vi "vPR_translate.vi"(9 "資料表欄位名稱":string[](array[string]), 10 "欄位數":i32, 11 "Input":T1(array[cluster])) -> (3 "輸出資料":string[][](array[string]))   [LabVIEW 2019]
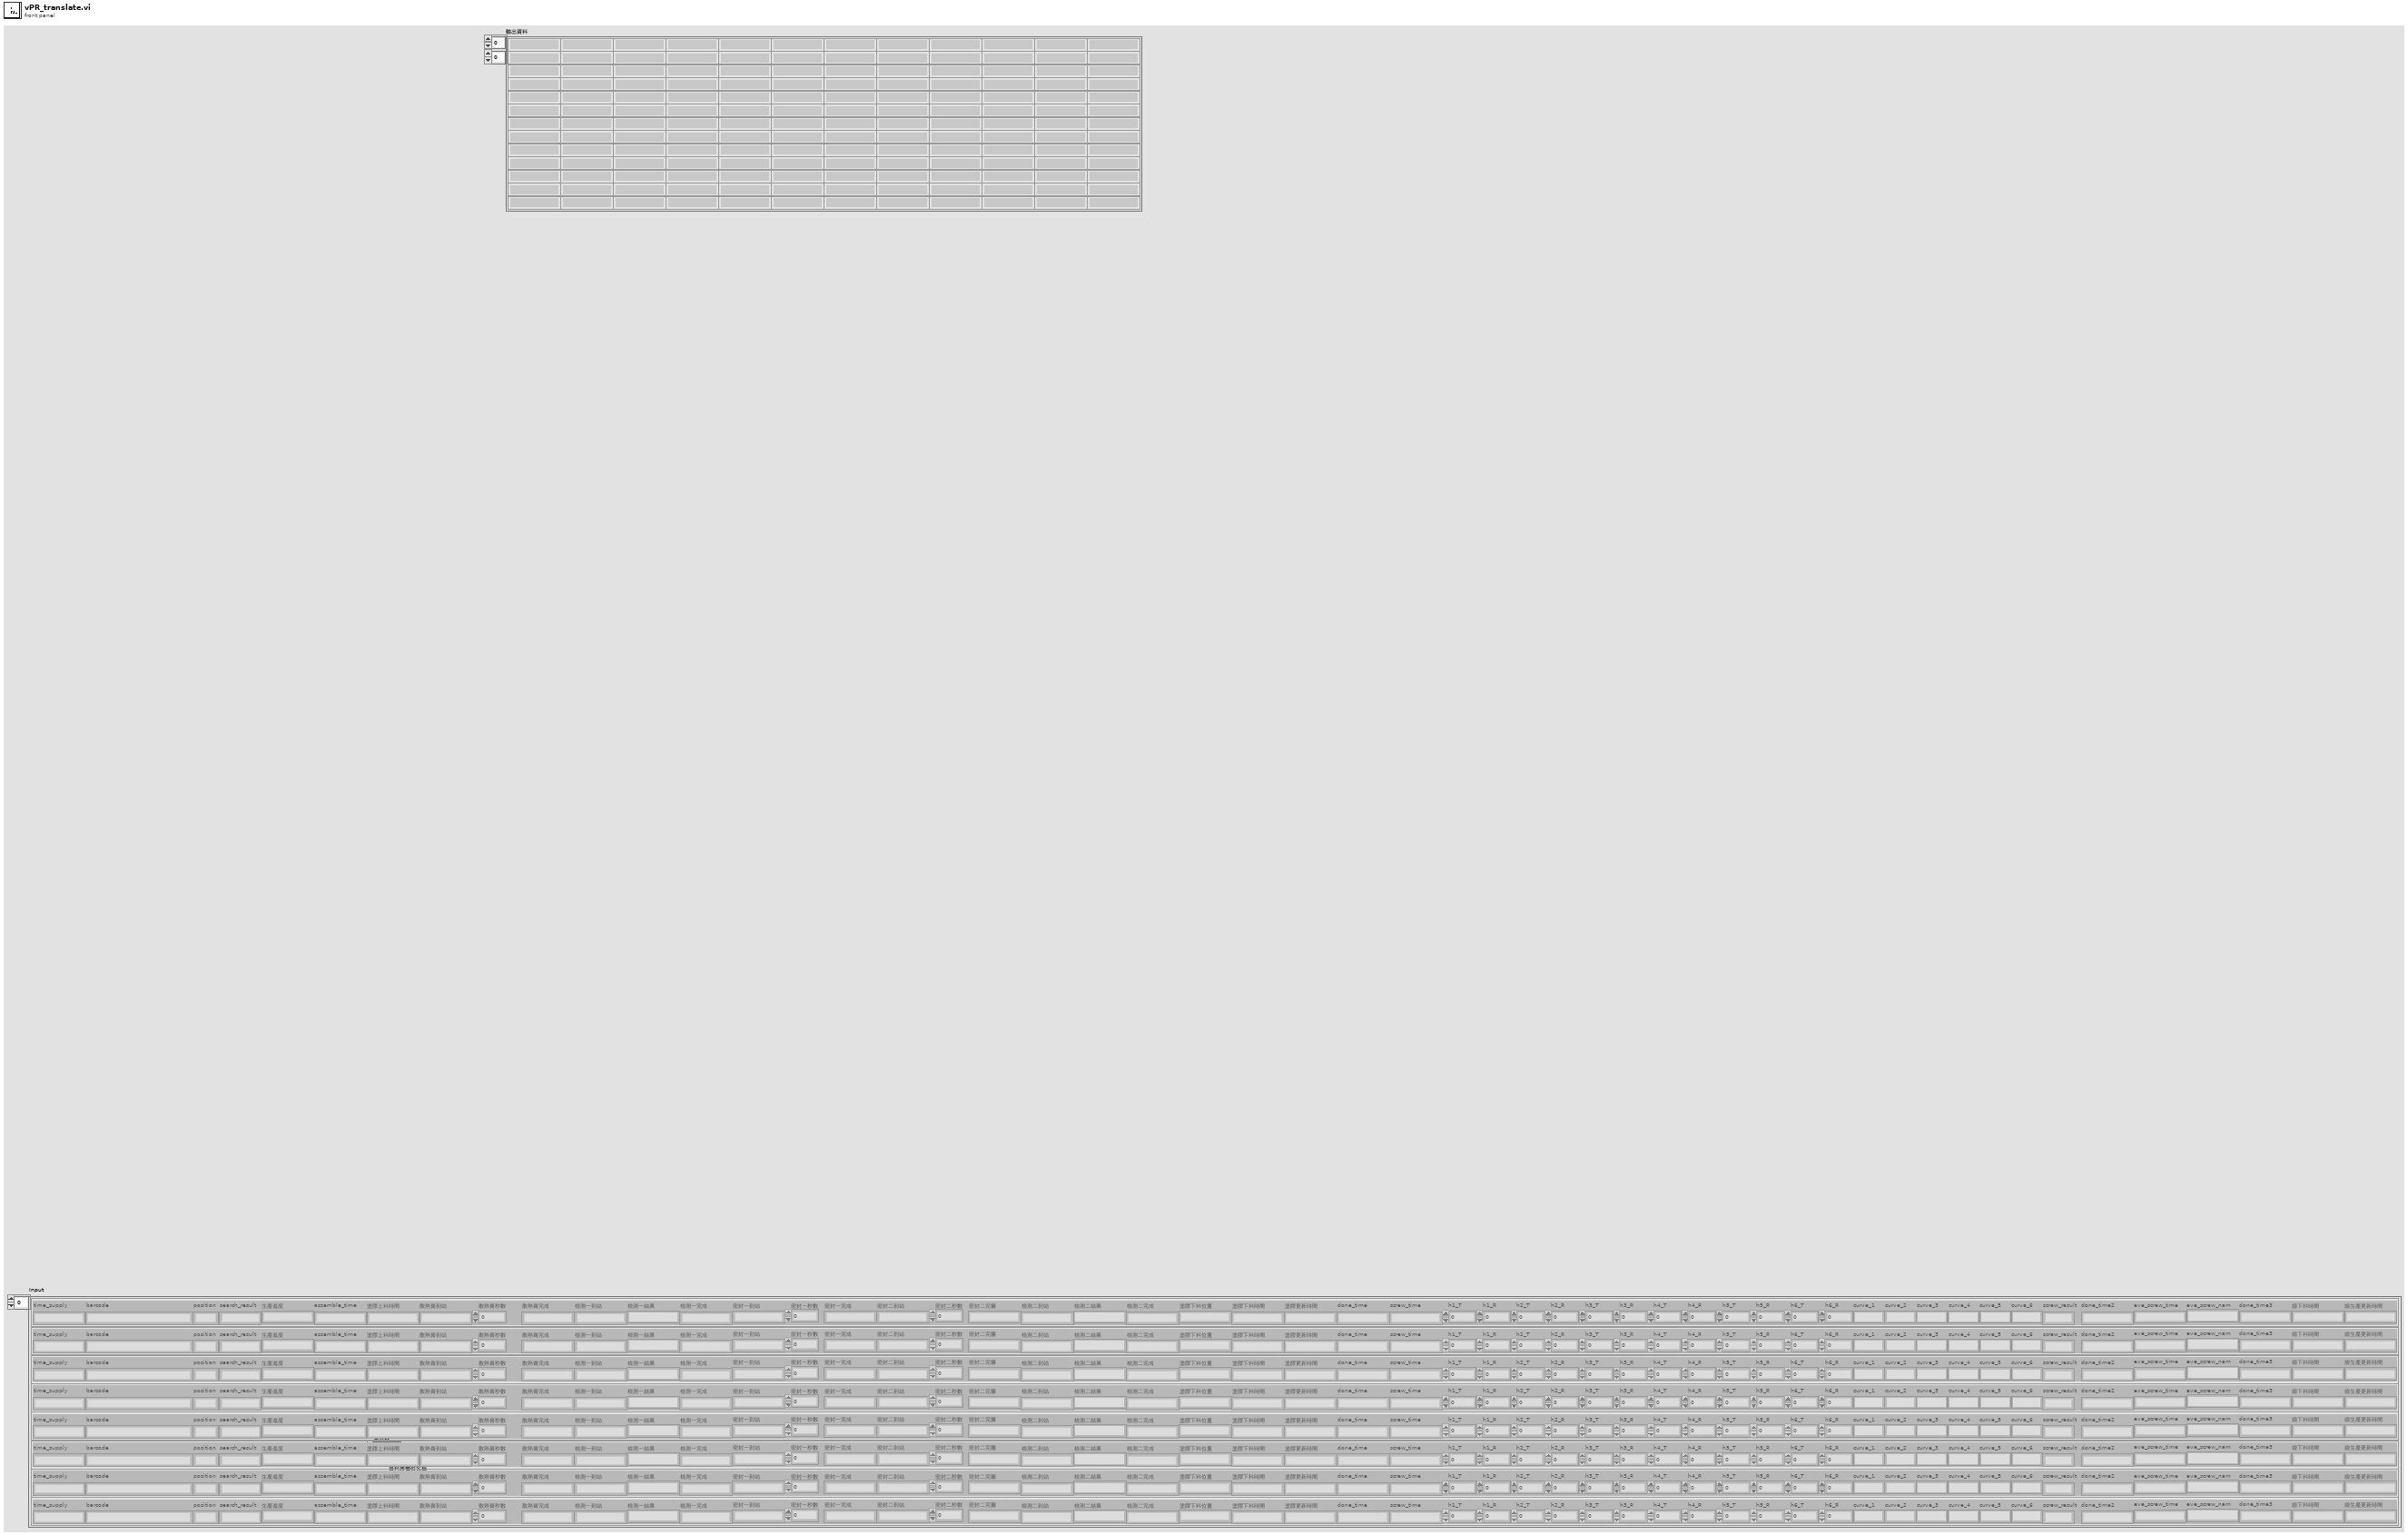
[diagram p1: front panel]
types:
  T1 = cluster{"time_supply":string, "barcode":string, "position":string, "search_result":string, "生產進度":string, "assemble_time":string, "塗膠上料時間":string, "散熱膏到站":string, "散熱膏秒數":dbl, "散熱膏完成":string, "檢測一到站":string, "檢測一結果":string, "檢測一完成":string, "密封一到站":string, "密封一秒數":dbl, "密封一完成":string, "密封二到站":string, "密封二秒數":dbl, "密封二完籌":string, "檢測二到站":string, "檢測二結果":string, "檢測二完成":string, "塗膠下料位置":string, "塗膠下料時間":string, "塗膠更新時間":string, "done_time":string, "screw_time":string, "h1_T":dbl, "h1_R":dbl, "h2_T":dbl, "h2_R":dbl, "h3_T":dbl, "h3_R":dbl, "h4_T":dbl, "h4_R":dbl, "h5_T":dbl, "h5_R":dbl, "h6_T":dbl, "h6_R":dbl, "curve_1":string, "curve_2":string, "curve_3":string, "curve_4":string, "curve_5":string, "curve_6":string, "screw_result":string, "done_time2":string, "eve_screw_time":string, "eve_screw_nam":string, "done_time3":string, "總下料時間":string, "總生產更新時間":string}[]
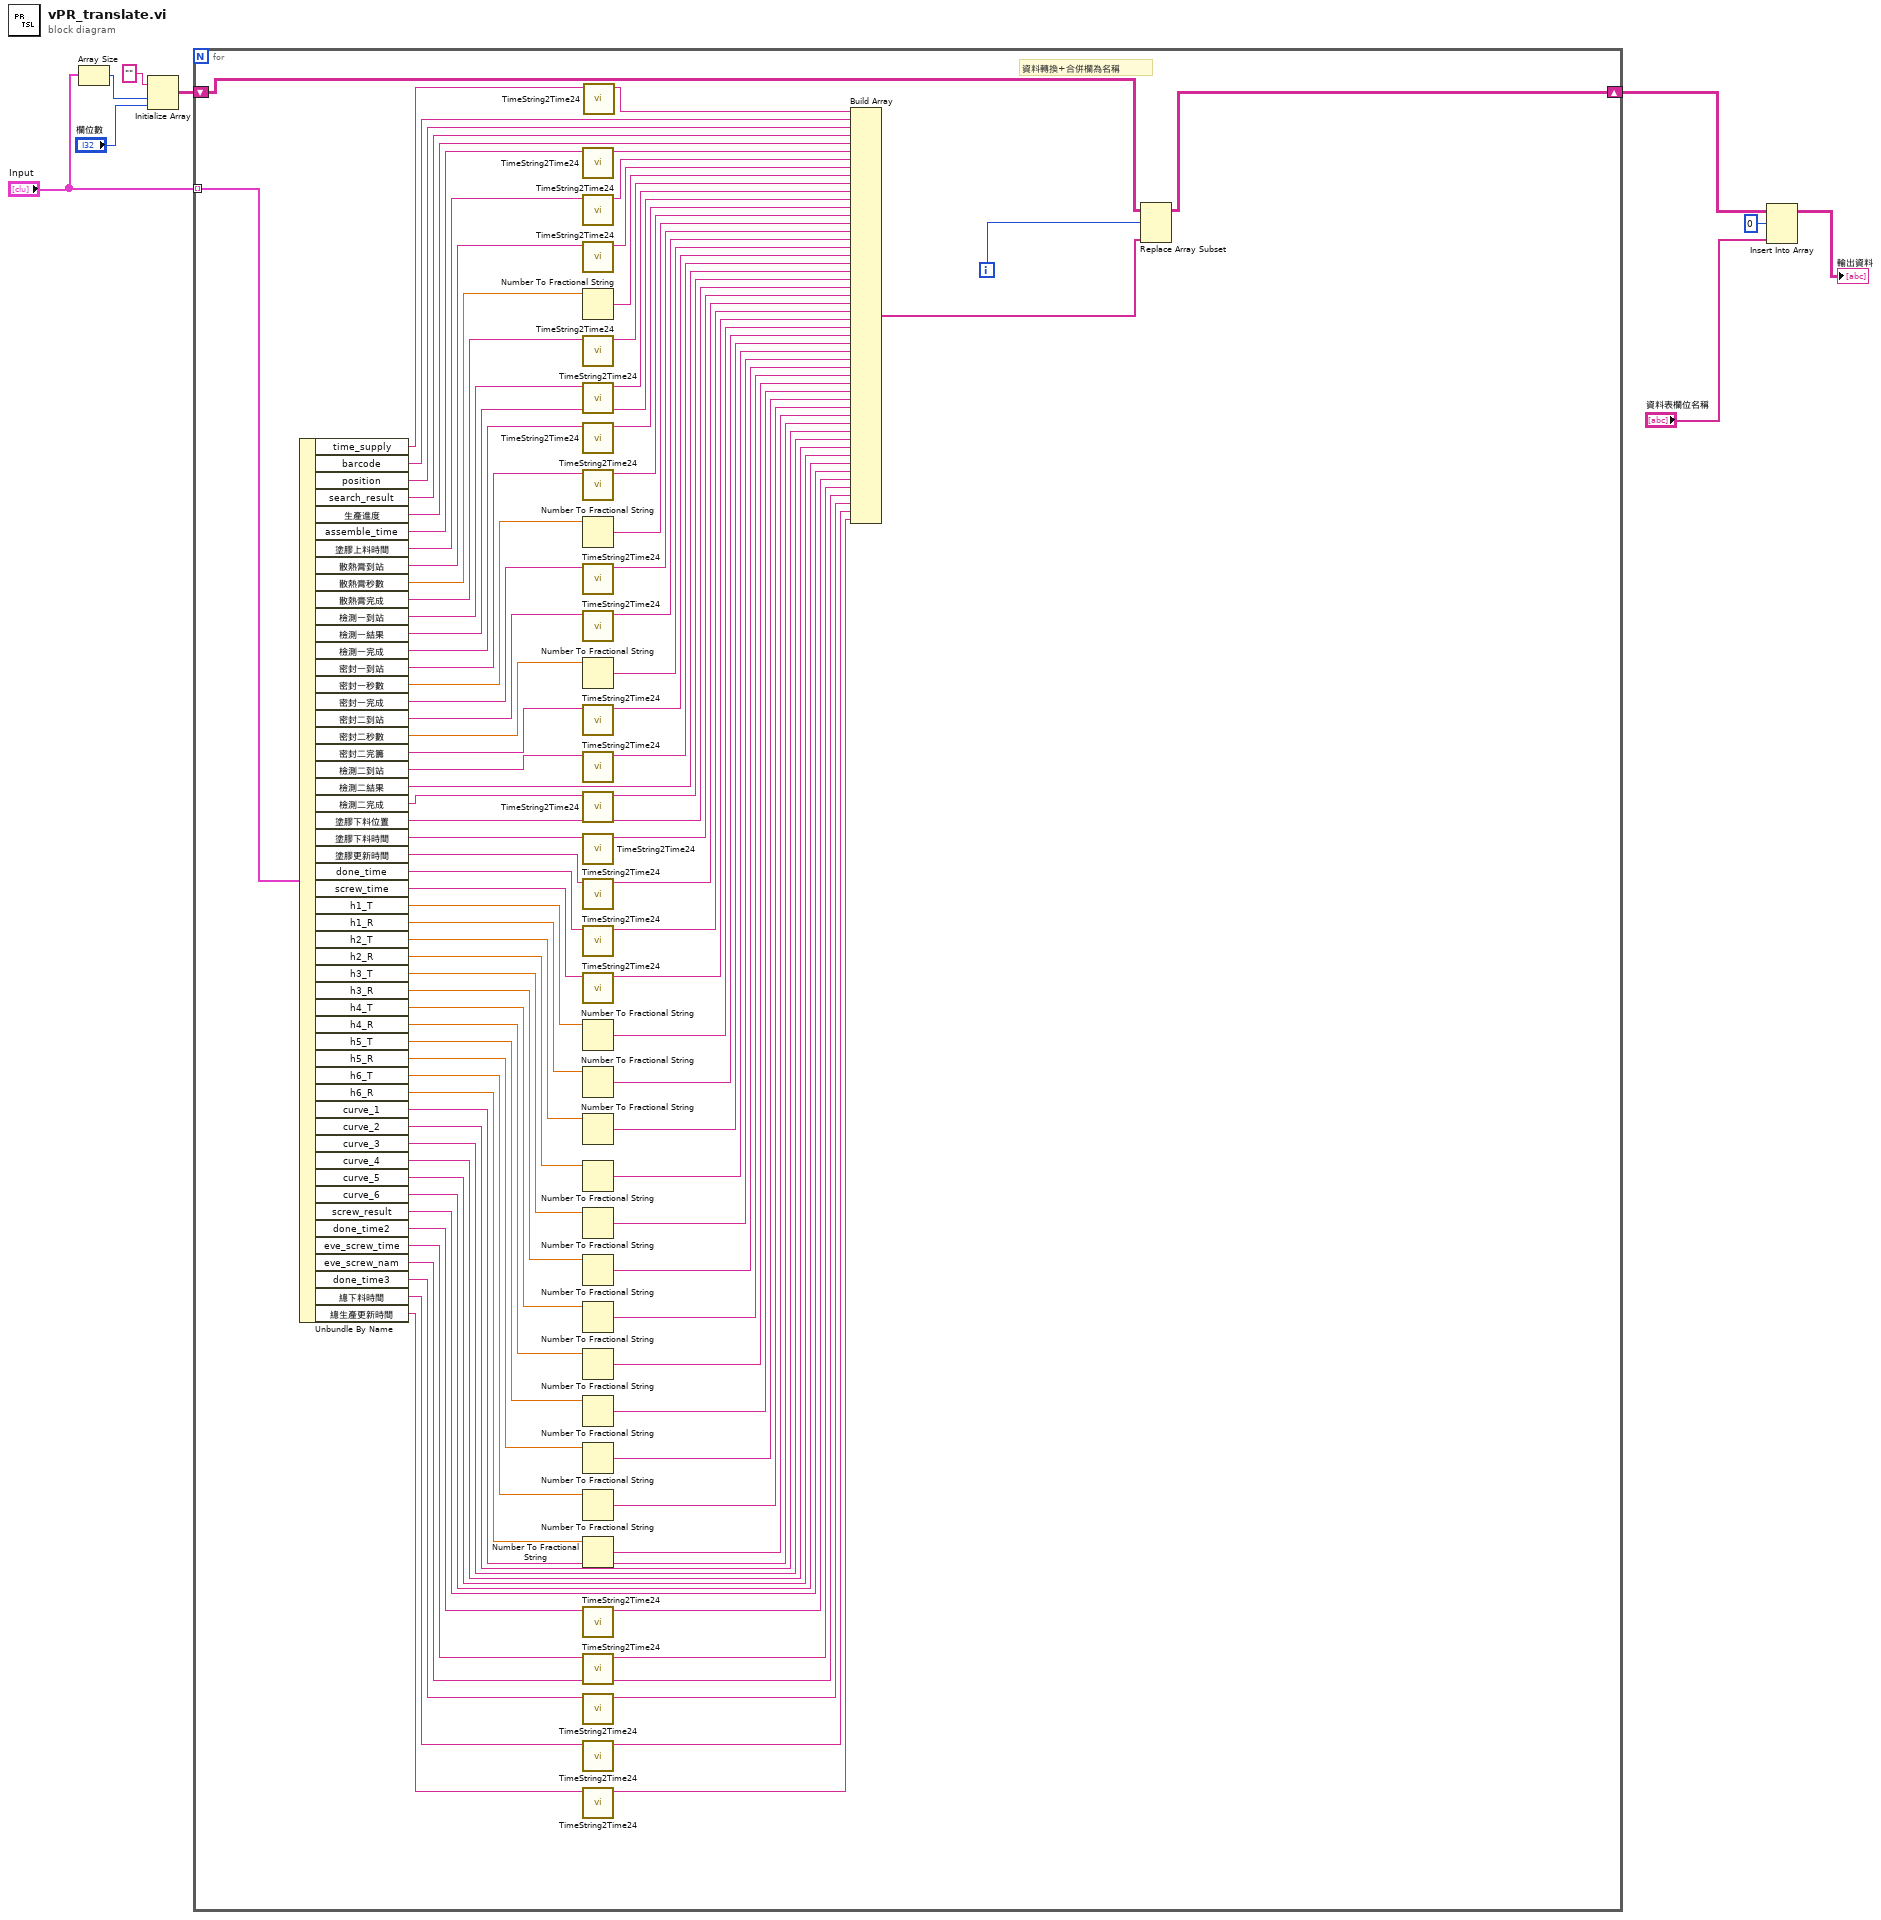
[diagram p0: block diagram]
diagram:
  n1 = Array Size(array="Input") -> (size(s)=w2:i32)
  n2 = Initialize Array("" ("element"), w2, "欄位數") -> (w5:string[][])
  n3 = for {
    tunnel: "Input" -> [w103] mode=indexing
    shift-right: [w99] -> w6
    shift-left: w5 -> [w102]
    i -> [w100]
    # "資料轉換+合併欄為名稱"
    n4 = Unbundle By Name(w103) -> ("time_supply"=w96:string, "barcode"=w98:string, "position"=w97:string, "search_result"=w94:string, "生產進度"=w93:string, "assemble_time"=w91:string, "塗膠上料時間"=w90:string, "散熱膏到站"=w88:string, "散熱膏秒數"=w86:dbl, "散熱膏完成"=w84:string, "檢測一到站"=w83:string, "檢測一結果"=w80:string, "檢測一完成"=w79:string, "密封一到站"=w77:string, "密封一秒數"=w75:dbl, "密封一完成"=w73:string, "密封二到站"=w71:string, "密封二秒數"=w69:dbl, "密封二完籌"=w67:string, "檢測二到站"=w65:string, "檢測二結果"=w63:string, "檢測二完成"=w62:string, "塗膠下料位置"=w60:string, "塗膠下料時間"=w59:string, "塗膠更新時間"=w57:string, "done_time"=w55:string, "screw_time"=w52:string, "h1_T"=w51:dbl, "h1_R"=w50:dbl, "h2_T"=w49:dbl, "h2_R"=w48:dbl, "h3_T"=w47:dbl, "h3_R"=w46:dbl, "h4_T"=w45:dbl, "h4_R"=w44:dbl, "h5_T"=w43:dbl, "h5_R"=w42:dbl, "h6_T"=w41:dbl, "h6_R"=w40:dbl, "curve_1"=w27:string, "curve_2"=w26:string, "curve_3"=w25:string, "curve_4"=w24:string, "curve_5"=w23:string, "curve_6"=w22:string, "screw_result"=w21:string, "done_time2"=w19:string, "eve_screw_time"=w18:string, "eve_screw_nam"=w16:string, "done_time3"=w15:string, "總下料時間"=w14:string, "總生產更新時間"=w13:string)
    n5 = call "TimeString2Time24.vi"("時間字串"=w91) -> ("date/time string"=w92:string)  [unwired: 9 in, 1 out]
    n6 = call "TimeString2Time24.vi"("時間字串"=w90) -> ("date/time string"=w89:string)  [unwired: 9 in, 1 out]
    n7 = call "TimeString2Time24.vi"("時間字串"=w88) -> ("date/time string"=w87:string)  [unwired: 9 in, 1 out]
    n8 = Number To Fractional String(number=w86) -> (F-format string=w85:string)  [unwired: 3 in]
    n9 = call "TimeString2Time24.vi"("時間字串"=w84) -> ("date/time string"=w81:string)  [unwired: 9 in, 1 out]
    n10 = call "TimeString2Time24.vi"("時間字串"=w83) -> ("date/time string"=w82:string)  [unwired: 9 in, 1 out]
    n11 = call "TimeString2Time24.vi"("時間字串"=w79) -> ("date/time string"=w78:string)  [unwired: 9 in, 1 out]
    n12 = call "TimeString2Time24.vi"("時間字串"=w77) -> ("date/time string"=w76:string)  [unwired: 9 in, 1 out]
    n13 = Number To Fractional String(number=w75) -> (F-format string=w74:string)  [unwired: 3 in]
    n14 = call "TimeString2Time24.vi"("時間字串"=w73) -> ("date/time string"=w72:string)  [unwired: 9 in, 1 out]
    n15 = call "TimeString2Time24.vi"("時間字串"=w71) -> ("date/time string"=w70:string)  [unwired: 9 in, 1 out]
    n16 = Number To Fractional String(number=w69) -> (F-format string=w68:string)  [unwired: 3 in]
    n17 = call "TimeString2Time24.vi"("時間字串"=w67) -> ("date/time string"=w66:string)  [unwired: 9 in, 1 out]
    n18 = call "TimeString2Time24.vi"("時間字串"=w65) -> ("date/time string"=w64:string)  [unwired: 9 in, 1 out]
    n19 = call "TimeString2Time24.vi"("時間字串"=w62) -> ("date/time string"=w61:string)  [unwired: 9 in, 1 out]
    n20 = call "TimeString2Time24.vi"("時間字串"=w59) -> ("date/time string"=w58:string)  [unwired: 9 in, 1 out]
    n21 = call "TimeString2Time24.vi"("時間字串"=w57) -> ("date/time string"=w56:string)  [unwired: 9 in, 1 out]
    n22 = call "TimeString2Time24.vi"("時間字串"=w55) -> ("date/time string"=w54:string)  [unwired: 9 in, 1 out]
    n23 = call "TimeString2Time24.vi"("時間字串"=w52) -> ("date/time string"=w53:string)  [unwired: 9 in, 1 out]
    n24 = Number To Fractional String(number=w51) -> (F-format string=w39:string)  [unwired: 3 in]
    n25 = Number To Fractional String(number=w50) -> (F-format string=w38:string)  [unwired: 3 in]
    n26 = Number To Fractional String(number=w49) -> (F-format string=w37:string)  [unwired: 3 in]
    n27 = Number To Fractional String(number=w48) -> (F-format string=w36:string)  [unwired: 3 in]
    n28 = Number To Fractional String(number=w47) -> (F-format string=w35:string)  [unwired: 3 in]
    n29 = Number To Fractional String(number=w46) -> (F-format string=w34:string)  [unwired: 3 in]
    n30 = Number To Fractional String(number=w45) -> (F-format string=w33:string)  [unwired: 3 in]
    n31 = Number To Fractional String(number=w44) -> (F-format string=w32:string)  [unwired: 3 in]
    n32 = Number To Fractional String(number=w43) -> (F-format string=w31:string)  [unwired: 3 in]
    n33 = Number To Fractional String(number=w42) -> (F-format string=w30:string)  [unwired: 3 in]
    n34 = Number To Fractional String(number=w41) -> (F-format string=w29:string)  [unwired: 3 in]
    n35 = Number To Fractional String(number=w40) -> (F-format string=w28:string)  [unwired: 3 in]
    n36 = call "TimeString2Time24.vi"("時間字串"=w19) -> ("date/time string"=w20:string)  [unwired: 9 in, 1 out]
    n37 = call "TimeString2Time24.vi"("時間字串"=w18) -> ("date/time string"=w17:string)  [unwired: 9 in, 1 out]
    n38 = call "TimeString2Time24.vi"("時間字串"=w15) -> ("date/time string"=w12:string)  [unwired: 9 in, 1 out]
    n39 = call "TimeString2Time24.vi"("時間字串"=w14) -> ("date/time string"=w11:string)  [unwired: 9 in, 1 out]
    n40 = call "TimeString2Time24.vi"("時間字串"=w13) -> ("date/time string"=w10:string)  [unwired: 9 in, 1 out]
    n41 = call "TimeString2Time24.vi"("時間字串"=w96) -> ("date/time string"=w95:string)  [unwired: 9 in, 1 out]
    n42 = Build Array(w95, w98, w97, w94, w93, w92, w89, w87, w85, w81, w82, w80, w78, w76, w74, w72, w70, w68, w66, w64, w63, w61, w60, w58, w56, w54, w53, w39, w38, w37, w36, w35, w34, w33, w32, w31, w30, w29, w28, w27, w26, w25, w24, w23, w22, w21, w20, w17, w16, w12, w11, w10) -> (w101:string[])
    n43 = Replace Array Subset(array=w102, new element=w101, index (row)=w100) -> (w99:string[][])  [unwired: 1 in]
  }
  n44 = Insert Into Array(array=w6, index (row)=0, new element="資料表欄位名稱") -> (→"輸出資料":string[][])  [unwired: 1 in]
